vi "Day 13-2.vi"() -> ()   [LabVIEW 2019, in "Day 13.lvlib"]
uses:
  Day 13.lvlib
panel:
  out "size(s)":i32[](array[numeric])
  out "Result":bool[][](array[boolean])
  out "Without fold":bool[][](array[boolean])
  out "coordenate":i32[](array[numeric])
  out "axis":string[](array[string])
  out "Points coordenates":i32[][](array[numeric])
  in  "String":string="797,352\n70,595\n1049,372\n887,710\n774,607\n581,348\n827,238\n341,1\n1295,858\n1017,854\n370,430\n937,465\n592,51\n604,850\n1169,766\n754,565\n577,28\n534,128\n925,119\n985,217\n917,522\n1275,64\n897,74\n239,723\n547,450\n1039,676\n606,158\n313,561\n1275,463\n513,352\n278,494\n634,436\n909,31\n480,176\n18,100\n417,807\n1250,882\n1158,485\n1158,24\n587,716\n112,68\n704,46\n887,632\n127,158\n706,32\n967,680\n922,523\n524,121\n579,499\n1268,654\n475,662\n20,516\n1073,843\n570,742\n89,415\n423,520\n11,219\n1125,784\n585,614\n1079,374\n768,826\n1216,840\n1014,719\n808,409\n95,683\n1221,418\n1111,460\n159,869\n1159,404\n5,395\n1295,410\n1111,879\n233,555\n156,238\n1166,660\n952,66\n289,651\n35,207\n723,716\n540,568\n542,826\n75,723\n175,852\n671,484\n565,759\n363,210\n621,602\n922,259\n293,152\n1287,348\n703,469\n1292,794\n1005,884\n423,268\n514,301\n862,800\n35,324\n219,864\n70,299\n800,611\n937,669\n187,236\n512,187\n464,810\n92,147\n5,445\n35,239\n233,339\n1275,324\n952,380\n360,267\n159,473\n1275,100\n530,375\n1061,171\n171,656\n1001,768\n648,861\n586,840\n1153,365\n1136,494\n800,283\n55,226\n1289,682\n1203,478\n763,444\n244,50\n401,31\n284,661\n1201,56\n1221,479\n239,781\n1049,522\n629,768\n25,451\n989,893\n224,329\n541,542\n68,168\n159,82\n962,660\n1169,234\n1026,849\n127,736\n50,131\n335,42\n745,639\n18,709\n547,478\n701,17\n975,852\n733,85\n70,747\n823,28\n89,476\n186,278\n329,229\n681,126\n206,849\n1238,145\n1101,684\n887,235\n897,820\n504,135\n141,128\n898,152\n673,819\n725,614\n537,333\n107,528\n1144,75\n652,656\n206,781\n510,611\n701,877\n363,684\n796,301\n120,576\n475,232\n1043,301\n694,382\n468,168\n1121,523\n341,721\n5,1\n251,753\n641,781\n704,158\n472,212\n952,175\n518,254\n17,712\n997,561\n1168,687\n1290,572\n102,341\n769,800\n54,250\n1183,417\n430,599\n1265,17\n271,39\n889,224\n87,723\n18,185\n565,387\n1043,794\n107,2\n179,232\n1078,392\n1174,196\n577,85\n5,51\n746,257\n867,649\n992,3\n1039,218\n117,882\n373,221\n922,399\n633,682\n519,268\n77,866\n100,886\n909,583\n510,548\n1221,415\n1186,519\n254,667\n846,278\n467,658\n306,719\n619,512\n1297,445\n776,128\n1275,431\n293,516\n405,723\n513,766\n361,264\n319,208\n423,632\n1034,651\n1292,548\n483,691\n1133,173\n426,553\n401,194\n724,597\n1285,451\n956,868\n423,626\n1256,644\n798,682\n488,75\n214,785\n937,429\n430,565\n1139,875\n20,458\n584,267\n1210,529\n226,857\n1069,820\n1216,54\n1084,37\n355,392\n370,799\n159,418\n997,51\n341,273\n1019,658\n827,19\n395,389\n552,151\n1263,469\n378,31\n467,796\n1272,512\n388,135\n1009,891\n661,144\n1144,819\n731,499\n405,843\n415,171\n87,611\n353,219\n637,819\n483,19\n743,723\n361,630\n75,171\n1099,693\n1077,339\n186,481\n925,215\n950,179\n1135,852\n541,352\n676,436\n616,382\n385,215\n141,234\n547,814\n370,213\n791,626\n775,187\n1151,812\n987,320\n212,774\n510,794\n291,158\n512,458\n1168,436\n763,864\n233,670\n373,673\n400,774\n1102,607\n284,337\n681,768\n1169,10\n724,54\n48,46\n981,665\n1305,472\n746,705\n964,182\n1183,736\n716,311\n226,275\n1151,418\n25,320\n1233,866\n1056,151\n947,210\n1044,75\n266,47\n109,56\n107,668\n1129,350\n348,10\n1260,315\n413,74\n1190,781\n964,570\n78,35\n956,250\n141,766\n276,651\n535,707\n1089,887\n1141,141\n189,523\n1044,819\n159,476\n800,100\n33,154\n1240,299\n318,891\n440,785\n1057,759\n1073,866\n376,95\n1014,66\n45,877\n703,425\n382,80\n846,250\n554,171\n565,59\n1285,574\n388,399\n636,100\n1203,416\n186,726\n962,98\n268,290\n358,66\n117,689\n835,438\n176,45\n45,17\n713,567\n1026,233\n271,666\n1014,842\n1232,35\n592,843\n1196,239\n934,95\n576,35\n1242,726\n354,250\n239,113\n171,19\n189,14\n1280,623\n842,413\n1240,267\n109,420\n306,175\n889,448\n740,742\n1190,576\n920,51\n910,774\n1059,753\n475,456\n522,724\n141,10\n1169,110\n554,843\n513,318\n977,638\n997,621\n1280,445\n73,311\n358,380\n1210,886\n477,273\n1151,476\n370,109\n977,893\n734,35\n423,710\n1088,10\n832,583\n537,176\n383,814\n843,684\n403,499\n1026,9\n468,413\n855,158\n728,145\n388,759\n109,26\n77,332\n1305,499\n383,855\n1280,604\n33,264\n470,660\n671,410\n893,807\n1073,807\n1241,280\n873,56\n674,633\n1232,411\n100,365\n691,830\n639,484\n895,171\n378,863\n1292,709\n142,207\n341,497\n50,602\n385,775\n512,660\n624,604\n1237,583\n343,662\n1069,522\n674,634\n838,212\n835,456\n354,644\n987,574\n187,348\n554,227\n1169,576\n109,474\n5,449\n955,502\n691,684\n293,488\n17,768\n570,152\n962,12\n281,127\n897,332\n1138,207\n475,438\n850,78\n634,567\n1139,238\n1218,747\n376,239\n100,456\n464,616\n536,287\n355,884\n825,499\n1262,400\n472,186\n882,37\n21,112\n1193,15\n634,458\n296,828\n870,785\n609,669\n1059,141\n587,178\n1151,82\n636,633\n305,884\n231,626\n565,863\n1044,707\n330,75\n905,275\n1201,474\n865,176\n937,673\n325,217\n82,50\n786,491\n1056,667\n84,600\n435,30\n346,261\n1124,278\n827,875\n586,493\n706,490\n783,288\n1026,213\n969,173\n35,548\n1017,488\n537,431\n800,794\n370,457\n1201,420\n791,420\n540,326\n1218,299\n815,389\n1039,855\n997,397\n25,443\n1098,774\n637,75\n651,768\n1168,682\n397,838\n77,85\n306,255\n269,663\n597,327\n825,589\n745,835\n18,794\n189,595\n1001,126\n643,219\n1304,413\n1223,723\n437,502\n100,723\n889,672\n1215,683\n1059,499\n1262,494\n1282,784\n870,557\n1102,287\n997,358\n893,87\n1032,494\n373,429\n387,301\n1237,642\n388,595\n535,187\n1288,660\n1046,51\n1093,838\n1044,495\n1084,619\n440,557\n1293,187\n346,570\n792,644\n413,332\n832,54\n1299,219\n383,666\n1044,135\n934,400\n763,814\n940,437\n661,445\n1026,337\n1305,445\n910,227\n682,308\n42,688\n370,95\n191,268\n1002,772\n343,214\n1210,723\n306,799\n1029,575\n738,844\n1290,119\n199,879\n485,395\n1228,50\n455,158\n157,365\n57,567\n1104,849\n1121,747\n1158,171\n1272,96\n78,411\n264,51\n539,89\n237,843\n979,499\n331,395\n1277,740\n445,210\n141,318\n94,54\n464,250\n991,686\n1260,131\n341,358\n142,212\n1169,128\n1056,326\n684,112\n949,264\n840,660\n733,361\n644,633\n57,119\n884,553\n341,536\n882,409\n1151,25\n30,333\n512,682\n47,425\n261,522\n1123,658\n686,604\n633,212\n706,315\n171,238\n950,627\n53,756\n1124,369\n1289,782\n313,273\n233,672\n2,432\n437,56\n141,576\n221,887\n564,705\n385,679\n576,859\n594,12\n1166,731\n1275,239\n770,326\n552,105\n278,400\n1124,616\n1123,236\n940,457\n976,481\n678,861\n1004,95\n1168,234\n662,861\n512,212\n1206,10\n284,457\n676,660\n1203,668\n211,693\n923,301\n800,548\n775,707\n1026,557\n922,495\n294,267\n370,437\n604,490\n1029,109\n181,350\n1119,268\n1086,329\n321,1\n666,633\n791,474\n691,64\n793,226\n1039,39\n428,37\n667,227\n358,445\n554,723\n689,602\n388,259\n400,227\n826,768\n20,322\n567,171\n1153,529\n301,798\n1168,484\n\nfold along x=655\nfold along y=447\nfold along x=327\nfold along y=223\nfold along x=163\nfold along y=111\nfold along x=81\nfold along y=55\nfold along x=40\nfold along y=27\nfold along y=13\nfold along y=6"
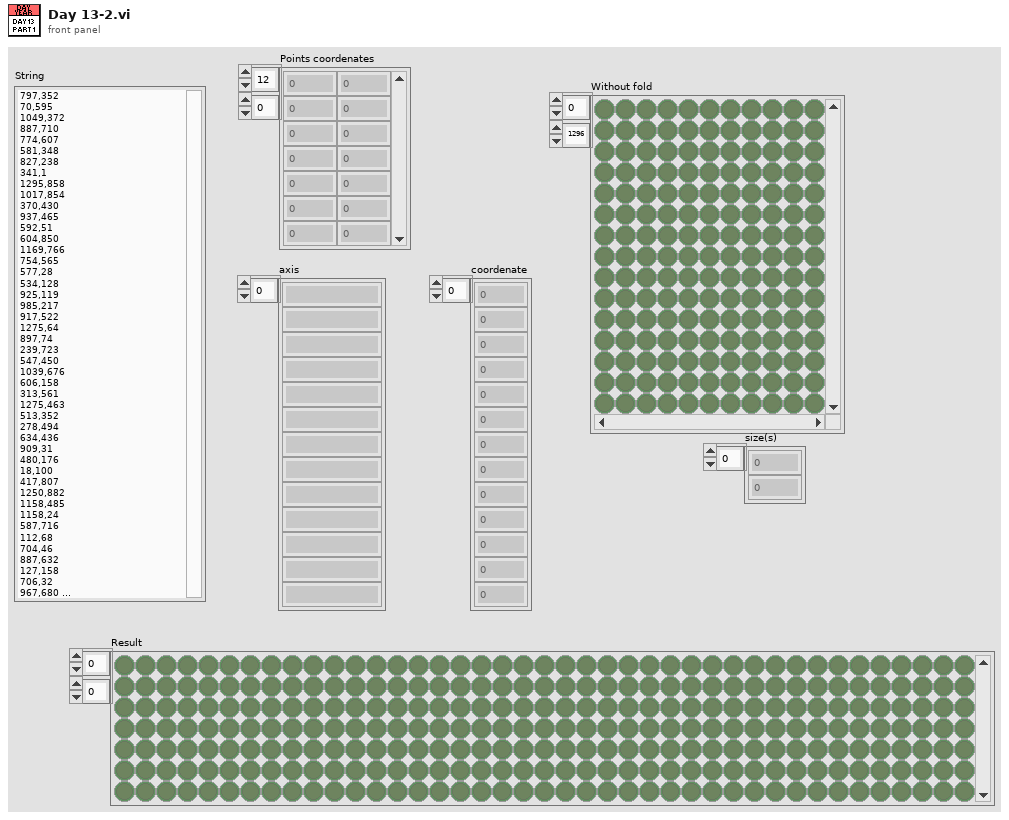
[diagram p1: front panel]
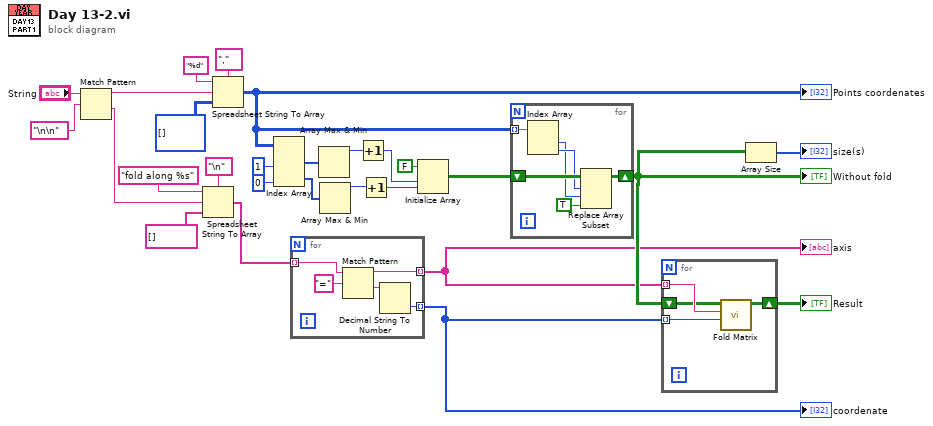
[diagram p0: block diagram]
diagram:
  n1 = Match Pattern(string="String", regular expression="\n\n") -> (before substring=w23:string, after substring=w18:string)  [unwired: 1 in, 2 out]
  n2 = Spreadsheet String To Array(delimiter (Tab)="\n", format string="fold along %s", spreadsheet string=w18, array type (2D Dbl)=string[] []) -> (array=w17:string[])
  n3 = Spreadsheet String To Array(delimiter (Tab)=",", format string="%d", spreadsheet string=w23, array type (2D Dbl)=i32[][] []) -> (array=w15:i32[][])
  "Points coordenates" <- w15
  n4 = Index Array(array=w15, index (col) #1=1 ("disabled index (col)"), index (col) #2=0 ("index (col)")) -> (element #1=w12:i32[], element #2=w11:i32[])  [unwired: 2 in]
  n5 = for {
    tunnel: w17 -> [w32] mode=indexing
    tunnel: [w29] -> w1 mode=indexing
    tunnel: [w28] -> w2 mode=indexing
    n6 = Match Pattern(string=w32, regular expression="=") -> (before substring=w28:string, after substring=w30:string)  [unwired: 1 in, 2 out]
    n7 = Decimal String To Number(string=w30) -> (number=w29:i32)  [unwired: 2 in, 1 out]
  }
  "axis" <- w2
  "coordenate" <- w1
  n8 = Array Max & Min(array=w12) -> (max value=w9:i32)  [unwired: 3 out]
  n9 = Array Max & Min(array=w11) -> (max value=w8:i32)  [unwired: 3 out]
  n10 = Increment(x=w9) -> (x+1=w6:i32)
  n11 = Increment(x=w8) -> (x+1=w7:i32)
  n12 = Initialize Array(FALSE, w6, w7) -> (w10:bool[][])
  n13 = for {
    tunnel: w15 -> [w37] mode=indexing
    shift-right: [w35] -> w4
    shift-left: w10 -> [w38]
    n14 = Index Array(array=w37) -> (element #1=w33:i32, element #2=w34:i32)  [unwired: 2 in]
    n15 = Replace Array Subset(array=w38, new element=TRUE ("new element/subarray"), index (row)=w34, index (col)=w33) -> (w35:bool[][])
  }
  "Without fold" <- w4
  n16 = for {
    tunnel: w2 -> [w42] mode=indexing
    tunnel: w1 -> [w41] mode=indexing
    shift-right: [w40] -> w5
    shift-left: w4 -> [w39]
    n17 = call "Fold Matrix.vi"("Index"=w41, "Coordenate"=w42, "Dots Matrix"=w39) -> ("Result"=w40:bool[][])  [unwired: 8 in]
  }
  "Result" <- w5
  n18 = Array Size(array=w4) -> (size(s)=→"size(s)":i32[])
